vi "Create Created.vi"(6 "Alias":string, 9 "Actor":refnum<class "Actor.lvclass">, 10 "Actor in":refnum<class "Actor.lvclass">) -> (0 "Error out":errorcluster, 2 "Actor out":refnum<class "Actor.lvclass">)   [LabVIEW 2025, in "jettl.lvlib" / "Actor.lvlib"]
uses:
  Actor.lvlib
  Actor/Actor.lvclass
  Error/Error.lvlib
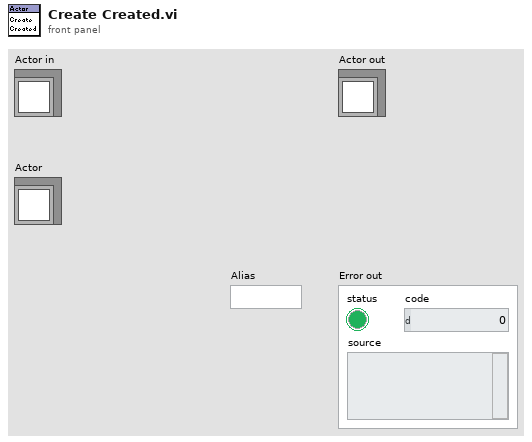
[diagram p1: front panel]
types:
  T1 = typedef "jettl.lvlib/Actor.lvlib/Created Aliases.ctl" = set{string}
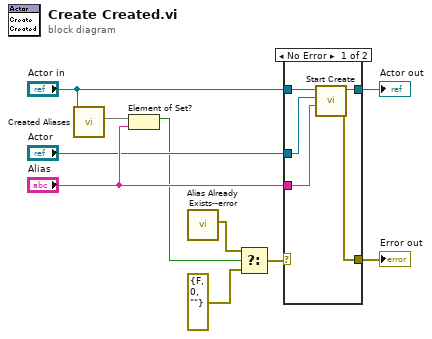
[diagram p0: block diagram]
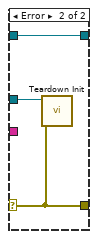
[diagram p2: hidden frame]
diagram:
  n1 = call-dynamic "Created Aliases.vi"("Actor in"="Actor in") -> ("Created Aliases"=w8:T1)  [unwired: 10 in]
  n2 = Element of Set?(10:"Alias", 11:w8) -> (3:w3:bool)
  n3 = call "Alias Already Exists--error.vi"() -> ("Error"=w4:errorcluster)  [unwired: 11 in]
  n4 = Select(t=w4, s=w3, f=errorcluster {"status"=FALSE, "code"=0, "source"=""}) -> (s? t:f=w1:errorcluster)
  n5 = case shown="No Error" w1 {
    selector: w1 -> [_ w16]
    tunnel: "Alias" -> [w11 _]
    tunnel: "Actor in" -> [w13 w18]
    tunnel: [w15 w16] -> w10
    tunnel: [w14 w18] -> w9
    tunnel: "Actor" -> [w12 w17]
    frame No Error {
      n6 = call-dynamic "Start Create.vi"("Alias"=w11, "Actor"=w12, "Actor in"=w13) -> ("Error out"=w15:errorcluster, "Actor out"=w14:refnum<class "Actor.lvclass">)  [unwired: 7 in]
    }
    frame Error {
      n7 = call-dynamic "Teardown Init.vi"("Error in"=w16, "Actor in"=w17) -> ()  [unwired: 10 in]
    }
  }
  "Error out" <- w10
  "Actor out" <- w9
